vi "Handle Events.vi"(8 "error in (no error)":errorcluster, 11 "TreeControlEventHandler":refnum<class "TreeControlEventHandler.lvclass">) -> ()   [LabVIEW 2015, in "ActorEvents.lvlib" / "TreeControlEventHandler.lvclass"]
uses:
  TreeControlEventHandler.lvclass
  IEventHandler/IEventHandler.lvclass
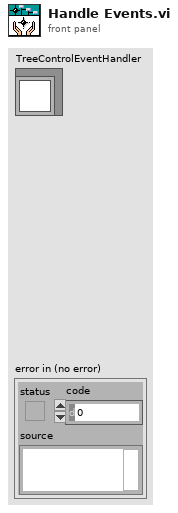
[diagram p1: front panel]
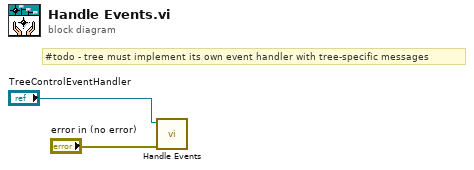
[diagram p0: block diagram]
diagram:
  # "#todo - tree must implement its own event handler with tree-specific messages"
  n1 = call-parent "Handle Events.vi"("error in (no error)"="error in (no error)", "EventHandler"="TreeControlEventHandler") -> ()  [unwired: 10 in]
